vi "Scans.vi"(1 "Time zero (sec)":timestamp, 2 "Queue in":T1(array[cluster]) {"Scan settings in queue" items=["Regular", "Inverted"]; "Time of the last scan (s)" format="%<%H:%M:%S>t"; "When did you stick it in?" format="%<%H:%M:%S>t"; "Time to next scan (s)" format="%<%H:%M:%S>t"; "Time in rig (s)" format="%<%H:%M:%S>t"}) -> (0 "Queue out":T1(array[cluster]) {"Scan settings in queue" items=["Regular", "Inverted"]; "Time of the last scan (s)" format="%<%H:%M:%S>t"; "When did you stick it in?" format="%<%H:%M:%S>t"; "Time to next scan (s)" format="%<%H:%M:%S>t"; "Time in rig (s)" format="%<%H:%M:%S>t"})   [LabVIEW 2011]
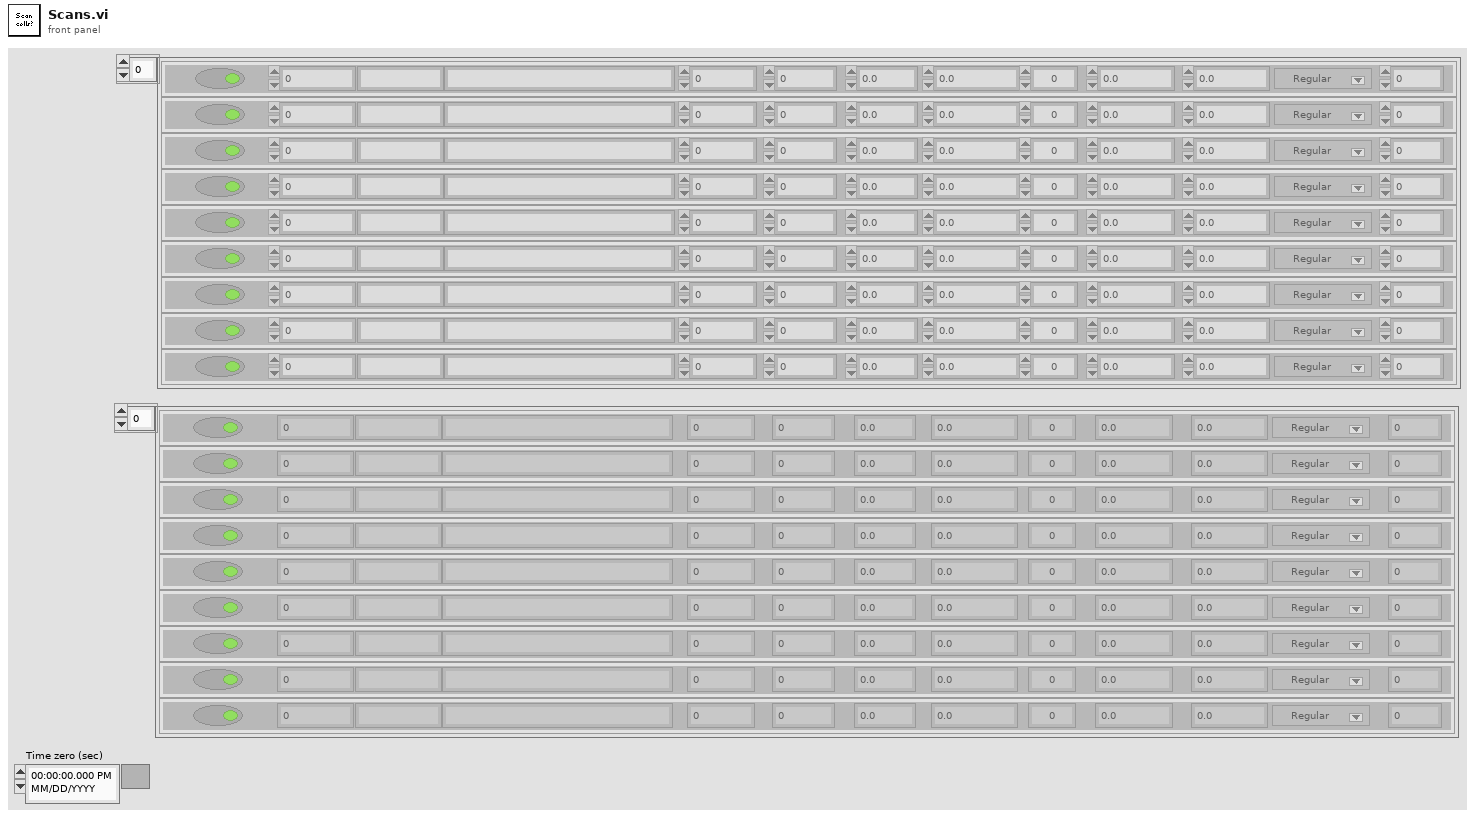
[diagram p1: front panel]
types:
  T1 = cluster{"Measure?":bool, "Area (cm^2)":dbl, "Cell Label":string, "Cell Description":string, "Cell Position":i32, "Time in rig (s)":dbl, "Time to next scan (s)":dbl, "Scan number":dbl, "When did you stick it in?":dbl, "Time between scans (s)":dbl, "Time of the last scan (s)":dbl, "Scan settings in queue":u16, "Sample Holder":dbl}[]
  T2 = cluster{"Measure?":bool, "Area (cm^2)":dbl, "Cell Label":string, "Cell Description":string, "Cell Position":i32, "Time in rig (s)":dbl, "Time to next scan (s)":dbl, "Scan number":dbl, "When did you stick it in?":dbl, "Time between scans (s)":dbl, "Time of the last scan (s)":dbl, "Scan settings in queue":u16, "Sample Holder":dbl}
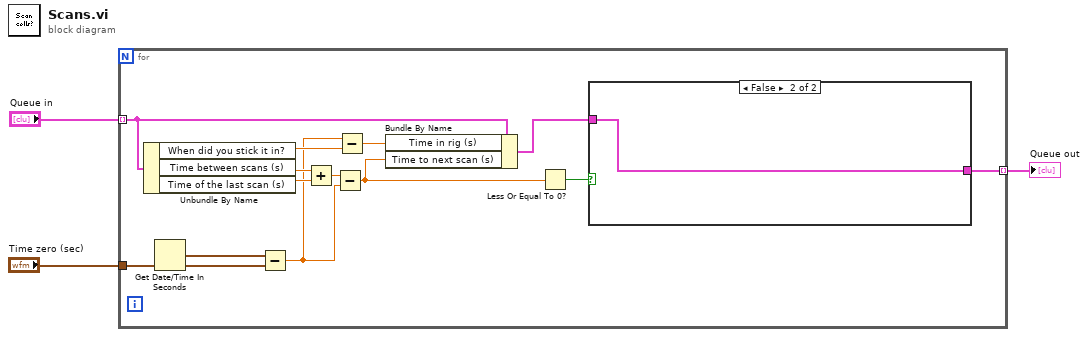
[diagram p0: block diagram]
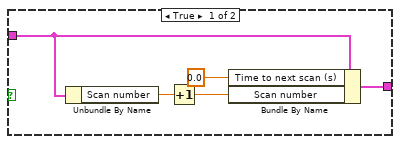
[diagram p2: hidden frame]
diagram:
  n1 = for {
    tunnel: "Time zero (sec)" -> [w15]
    tunnel: "Queue in" -> [w12] mode=indexing
    tunnel: [w13] -> w1 mode=indexing
    n2 = Unbundle By Name(w12) -> ("When did you stick it in?"=w10:dbl, "Time between scans (s)"=w8:dbl, "Time of the last scan (s)"=w9:dbl)
    n3 = Get Date/Time In Seconds() -> (seconds since 1Jan1904=w16:timestamp)
    n4 = Subtract(x=w16, y=w15) -> (x-y=w6:dbl)
    n5 = Add(x=w8, y=w9) -> (x+y=w7:dbl)
    n6 = Subtract(x=w7, y=w6) -> (x-y=w4:dbl)
    n7 = Subtract(x=w6, y=w10) -> (x-y=w5:dbl)
    n8 = Bundle By Name(cluster=w12, "Time in rig (s)"=w5, "Time to next scan (s)"=w4) -> (w11:T2)
    n9 = Less Or Equal To 0?(x=w4) -> (x <= 0?=w14:bool)
    n10 = case shown="False" w14 {
      tunnel: w11 -> [w18 w22]
      tunnel: [w21 w22] -> w13
      frame True {
        n11 = Unbundle By Name(w18) -> ("Scan number"=w17:dbl)
        n12 = Increment(x=w17) -> (x+1=w20:dbl)
        n13 = Bundle By Name(cluster=w18, "Time to next scan (s)"=0.0 ("Time since last scan (min)"), "Scan number"=w20) -> (w21:T2)
      }
      frame False {
      }
    }
  }
  "Queue out" <- w1
